vi "script debug.vi"() -> ()   [LabVIEW 2019]
uses:
  <vilib>/Utility/file.llb/Read Delimited Spreadsheet (DBL).vi
panel:
  out "all rows":dbl[][](array[numeric])
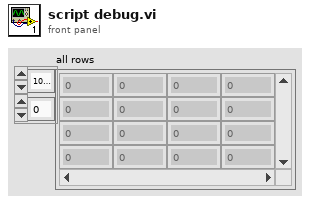
[diagram p1: front panel]
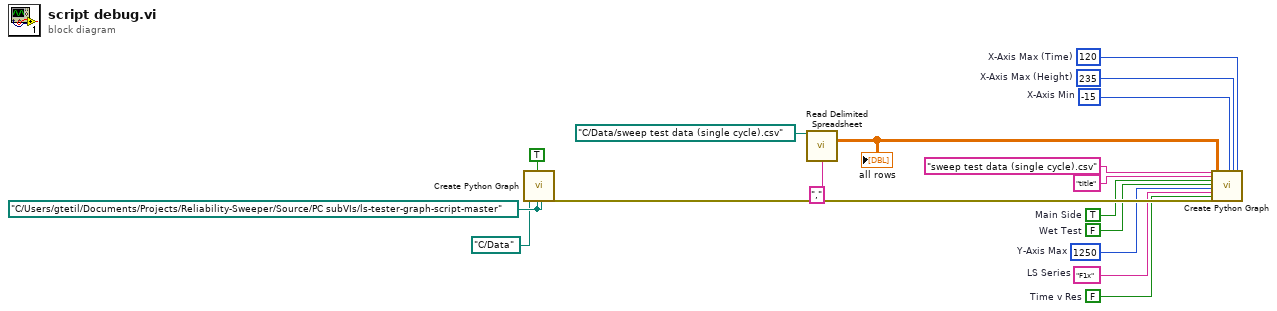
[diagram p0: block diagram]
diagram:
  w3 = 120  # X-Axis Max (Time)
  w4 = 235  # X-Axis Max (Height)
  w5 = -15  # X-Axis Min
  w6 = FALSE  # Time v Res
  w7 = "F1x"  # LS Series
  w8 = 1250  # Y-Axis Max
  w9 = FALSE  # Wet Test
  w10 = TRUE  # Main Side
  w11 = path "C:/Users/gtetil/Documents/Projects/Reliability-Sweeper/Source/PC subVIs/ls-tester-graph-script-master" ("Tolerances Path")
  n1 = call "Create Python Graph.vi"("Data Base Path"=path "C:/Data", "Init (F)"=TRUE, "Tolerances Path"=w11, "Python Script Directory"=w11) -> ("Error OUT"=w12:errorcluster)  [unwired: 23 in]
  n2 = call-poly <vilib>:"Read Delimited Spreadsheet.vi"("file path (dialog if empty)"=path "C:/Data/sweep test data (single cycle).csv", "delimiter (\\t)"="," ("delimiter (\\t)")) -> ("all rows"=w16:dbl[][])  [unwired: 8 in, 5 out]
  "all rows" <- w16
  n3 = call "Create Python Graph.vi"("File Name"="sweep test data (single cycle).csv", "Title"="title", "Main Side"=w10, "Wet Test"=w9, "Y-Axis Max"=w8, "LS Series"=w7, "Time v Res"=w6, "Error IN"=w12, "Data"=w16, "X-Axis Min"=w5, "X-Axis Max (Height)"=w4, "X-Axis Max (Time)"=w3) -> ()  [unwired: 15 in, 1 out]
